vi "Initialize.vi"(8 "error in (no error)":errorcluster, 10 "Zenoh Configuration":T1={"Configuration (file or JSON)"="", "Liveliness"=TRUE, "Liveliness Name"="", "Storage Key Expressions"=[]}, 11 "Zenoh in":refnum<class "Zenoh.lvclass">) -> (0 "error out":errorcluster, 3 "Zenoh out":refnum<class "Zenoh.lvclass">)   [LabVIEW 2021, in "Zenoh.lvclass"]
doc: "Initialize and open a Zenoh session. \nThe configuration JSON is a standard Zenoh configuration file. https://zenoh.io/docs/manual/configuration/\nLiveliness will allow tracking node status.\nThe Liveliness name can provide a specific name. If left blank the hostname-ipaddresses will be used.\n\nThe storage key expression (KE) used when creating an in-memory storage."
uses:
  Zenoh.lvclass
  typedef/Zenoh Configuration.ctl
  Zenoh.lvclass/Zenoh.ctl
  <vilib>/CIF Foundation/CIF Utilities/Networking/Networking_CIF_U.lvlib
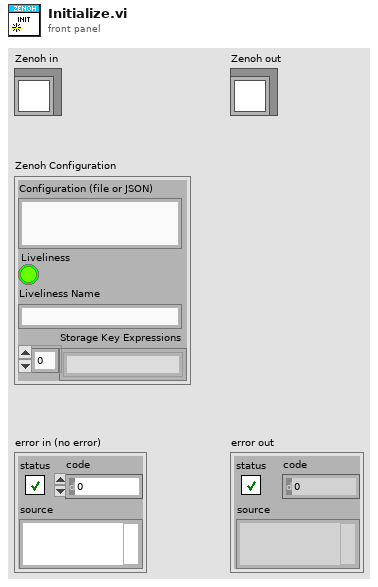
[diagram p1: front panel]
types:
  T1 = typedef "Zenoh.lvclass/Zenoh Configuration.ctl" = cluster{"Configuration (file or JSON)":string, "Liveliness":bool, "Liveliness Name":string, "Storage Key Expressions":string[]}
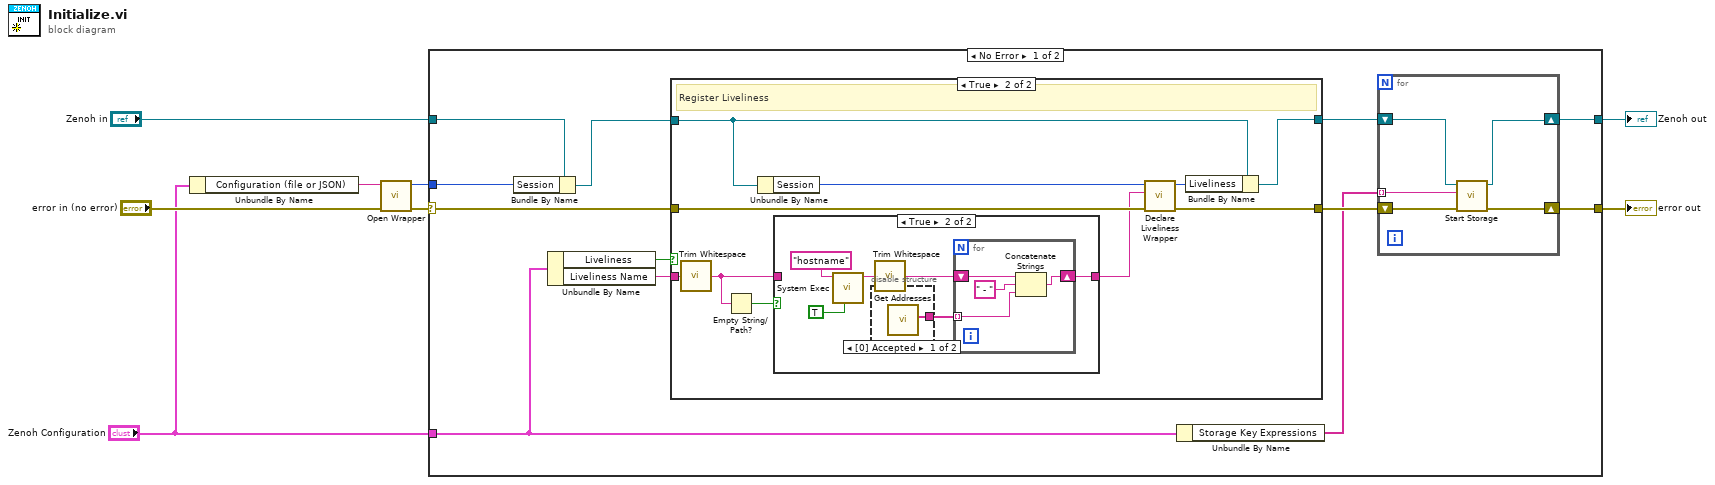
[diagram p0: block diagram]
diagram:
  n1 = Unbundle By Name("Zenoh Configuration") -> ("Configuration (file or JSON)"=w1:string)
  n2 = call "Open Wrapper.vi"("error in (no error)"="error in (no error)", "Configuration Json"=w1) -> ("error out"=w4:errorcluster, "Session"=w3:u64)  [unwired: 8 in]
  n3 = case shown="No Error" w4 {
    selector: w4 -> [w20 w51]
    tunnel: [w9 w51] -> w8
    tunnel: [w10 w50] -> w6
    tunnel: "Zenoh in" -> [w18 w50]
    tunnel: w3 -> [w17 _]
    tunnel: "Zenoh Configuration" -> [w12 _]
    frame No Error {
      n4 = Bundle By Name(cluster=w18, "Session"=w17) -> (w15:refnum<class "Zenoh.lvclass">)
      n5 = Unbundle By Name(w12) -> ("Liveliness"=w16:bool, "Liveliness Name"=w19:string)
      n6 = case shown="True" w16 {
        tunnel: w20 -> [w26 w37]
        tunnel: [w26 w36] -> w14
        tunnel: w19 -> [_ w32]
        tunnel: w15 -> [w27 w29]
        tunnel: [w27 w28] -> w13
        frame False {
          # "Don't Register Liveliness"
        }
        frame True {
          # "Register Liveliness"
          n7 = call <vilib>:"Trim Whitespace.vi"("string"=w32) -> ("trimmed string"=w34:string)  [unwired: 1 in]
          n8 = Empty String/Path?(string/path=w34) -> (empty?=w35:bool)
          n9 = Unbundle By Name(w29) -> ("Session"=w31:u64)
          n10 = case shown="True" w35 {
            tunnel: w34 -> [w38 _]
            tunnel: [w38 w40] -> w33
            frame False {
            }
            frame True {
              n11 = call <vilib>:"System Exec.vi"("run minimized? (F)"=TRUE, "command line"="hostname") -> ("standard output"=w43:string)  [unwired: 6 in, 3 out]
              n12 = disable-structure shown="[0] Accepted" {
                disable-tunnel: [w45 _] -> w39
                frame Enabled {
                  n13 = call <vilib>:"Get Addresses.vi"() -> ("Addresses"=w45:string[])  [unwired: 10 in, 1 out]
                }
                frame Disabled {
                }
              }
              n14 = call <vilib>:"Trim Whitespace.vi"("string"=w43) -> ("trimmed string"=w41:string)  [unwired: 1 in]
              n15 = for {
                shift-right: [w48] -> w40
                shift-left: w41 -> [w49]
                tunnel: w39 -> [w47] mode=indexing
                n16 = Concatenate Strings(w49, " - " ("string"), w47) -> (w48:string)
              }
            }
          }
          n17 = call "Declare Liveliness Wrapper.vi"("error in (no error)"=w37, "Key Expression"=w33, "Session in"=w31) -> ("error out"=w36:errorcluster, "Liveliness Token"=w30:u64)  [unwired: 7 in]
          n18 = Bundle By Name(cluster=w29, "Liveliness"=w30) -> (w28:refnum<class "Zenoh.lvclass">)
        }
      }
      n19 = Unbundle By Name(w12) -> ("Storage Key Expressions"=w11:string[])
      n20 = for {
        shift-right: [w22] -> w9
        shift-left: w14 -> [w25]
        shift-right: [w23] -> w10
        shift-left: w13 -> [w24]
        tunnel: w11 -> [w21] mode=indexing
        n21 = call "Start Storage.vi"("error in (no error)"=w25, "Storage Key Expression"=w21, "Zenoh in"=w24) -> ("error out"=w22:errorcluster, "Zenoh out"=w23:refnum<class "Zenoh.lvclass">)  [unwired: 7 in]
      }
    }
    frame Error {
    }
  }
  "error out" <- w8
  "Zenoh out" <- w6
